vi "z closure matching status call.vi"(8 "error in (no error)":errorcluster, 10 "mathing_status":cluster{"matching":bool}, 11 "closure":cluster{}) -> (0 "error out":errorcluster)   [LabVIEW 2021, in "zenohc.lvlib"]
doc: "void z_closure_matching_status_call(const struct z_loaned_closure_matching_status_t *closure,\n const struct z_matching_status_t *mathing_status);"
uses:
  zenohc.lvlib
  zenohc.dll
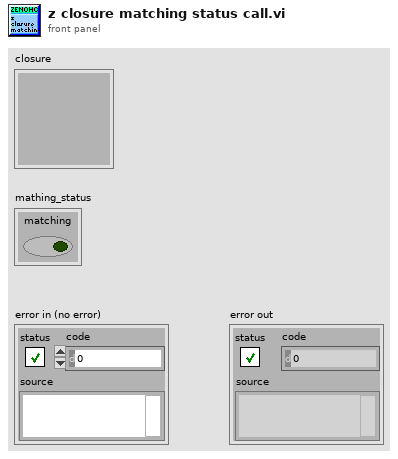
[diagram p1: front panel]
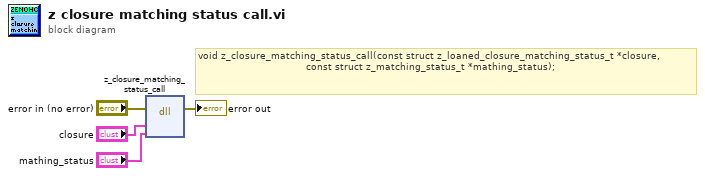
[diagram p0: block diagram]
diagram:
  # "void z_closure_matching_status_call(const struct z_loaned_closure_matching_status_t *closure,\n                                    const struct z_matching_status_t *mathing_status);"
  n1 = dll-call lib="D:/dev/zenoh_labview/zenohc/zenohc.*" fn="z_closure_matching_status_call"(error in="error in (no error)", "closure"="closure", "mathing_status"="mathing_status") -> (error out=→"error out":errorcluster)  [unwired: 5 in, 1 out]
